vi "get_average_laser_power.vi"(0 "Laser Power Q":T2, 1 "Cancel Notifier":T1, 2 "Averaging Time /s":u32, 11 "Error in":errorcluster) -> (4 "Laser Power Q Out":T2, 13 "Average Power / J":dbl, 15 "Error out":errorcluster)   [LabVIEW 2023]
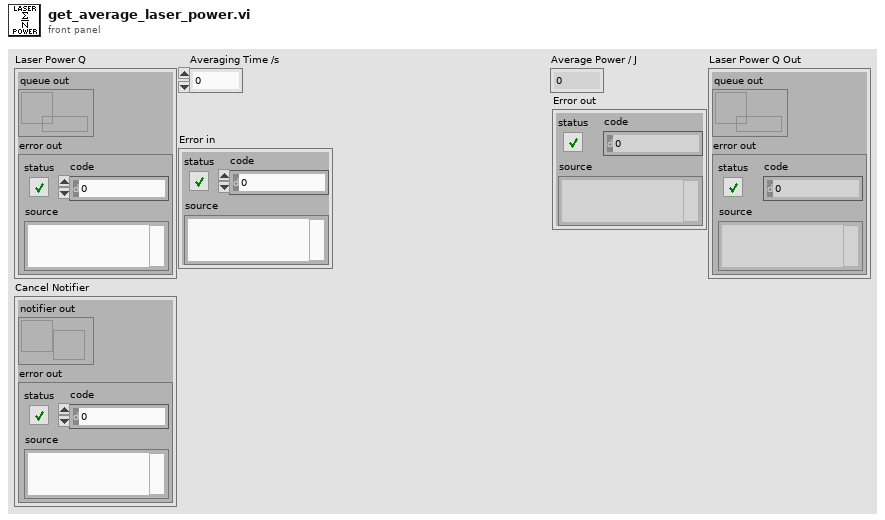
[diagram p1: front panel]
types:
  T1 = cluster{"notifier out":refnum<notifier>, "error out":errorcluster}
  T2 = cluster{"queue out":refnum<queue>, "error out":errorcluster}
  T3 = cluster{"Power Reading ":dbl, "T imestamp":dbl, "Status":i32}
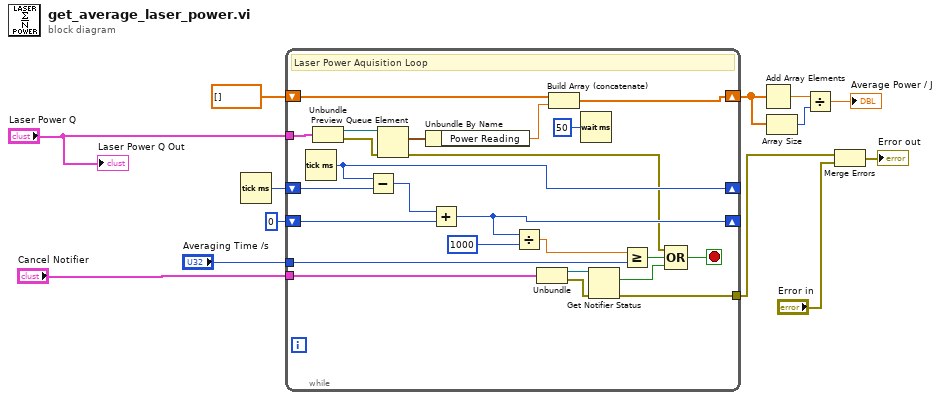
[diagram p0: block diagram]
diagram:
  n1 = Tick Count (ms)() -> (millisecond timer value=w11:u32)
  n2 = while {
    tunnel: "Laser Power Q" -> [w37]
    shift-right: [w30] -> w8
    shift-left: dbl[] [] -> [w32]
    shift-right: [w28] -> _
    shift-left: w11 -> [w29]
    shift-right: [w25] -> _
    shift-left: u32 0 -> [w26]
    tunnel: "Averaging Time /s" -> [w22]
    tunnel: "Cancel Notifier" -> [w19]
    tunnel: [w14] -> w1
    stop <- w20 stop-if-true
    # "Laser Power Aquisition Loop"
    n3 = Tick Count (ms)() -> (millisecond timer value=w28:u32)
    n4 = Unbundle(w37) -> ("queue out"=w36:refnum<queue>, "error out"=w35:errorcluster)
    n5 = Subtract(x=w28, y=w29) -> (x-y=w27:u32)
    n6 = Preview Queue Element(queue=w36, error in (no error)=w35) -> (element=w34:T3, error out=w15:errorcluster)  [unwired: 1 in, 2 out]
    n7 = Unbundle By Name(w34) -> ("Power Reading"=w33:dbl)
    n8 = Add(x=w27, y=w26) -> (x+y=w25:u32)
    n9 = Divide(x=w25, y=u32 1000) -> (x/y=w23:dbl)
    n10 = Unbundle(w19) -> ("notifier out"=w17:refnum<notifier>, "error out"=w16:errorcluster)
    n11 = Build Array (concatenate)(w32, w33) -> (w30:dbl[])
    n12 = Wait (ms)(milliseconds to wait=u32 50) -> ()  [unwired: 1 out]
    n13 = Get Notifier Status(notifier=w17, error in (no error)=w16) -> (current notification=w18:bool, error out=w14:errorcluster)  [unwired: 3 out]
    n14 = Greater Or Equal?(x=w23, y=w22) -> (x >= y?=w21:bool)
    n15 = Compound Arithmetic op=OR(w15, w21, w18) -> (w20:bool)
  }
  n16 = Add Array Elements(numeric array=w8) -> (sum=w9:dbl)
  n17 = Array Size(array=w8) -> (size(s)=w7:i32)
  n18 = Divide(x=w9, y=w7) -> (x/y=→"Average Power / J":dbl)
  n19 = Merge Errors(w1, "Error in") -> (→"Error out":errorcluster)
  "Laser Power Q Out" <- "Laser Power Q"
